vi "HEWH Check For Element Off During Normal Draw.vi"(6 "End of Draw Comparison":bool[][](array[boolean]), 9 "Test Complete":bool, 10 "Debug":bool, 11 "Power State":T1) -> (3 "Cutout after Test Complete":bool, 4 "End of Draw Comparison Output":bool[][](array[boolean]))   [LabVIEW 2023]
uses:
  Type Definitions/HEWH Power Elements.ctl
  Utility/Type Definitions/UTILITY Notifier.ctl
panel:
  out "Index Stop":i32
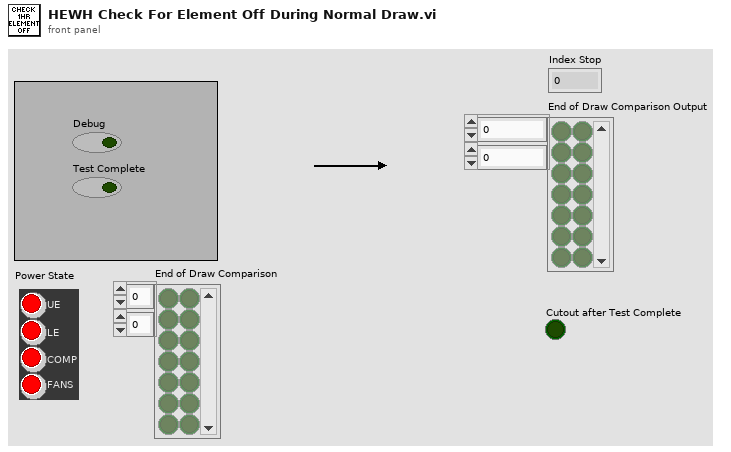
[diagram p1: front panel]
types:
  T1 = typedef "HEWH Power Elements.ctl" = cluster{"UE":bool, "LE":bool, "COMP":bool, "FANS":bool}
  T2 = typedef "UTILITY Notifier.ctl" = enum16{"Set", "Read", "Release Ref"}
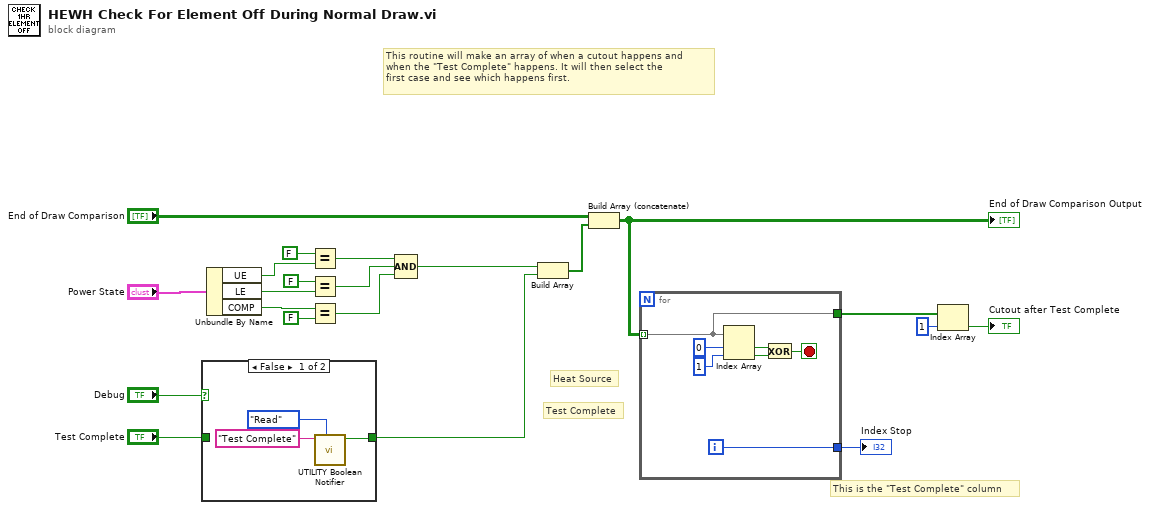
[diagram p0: block diagram]
diagram:
  # "Test Complete"
  # "Heat Source"
  # "This routine will make an array of when a cutout happens and \nwhen the \"Test Complete\" happens. It will then select the \nfirst case and see which happens first."
  # "This is the \"Test Complete\" column"
  n1 = case shown="False" "Debug" {
    tunnel: [w22 w25] -> w10
    tunnel: "Test Complete" -> [_ w25]
    frame False {
      n2 = call "UTILITY Boolean Notifier.vi"("Status"=UTILITY_Notifier."Read", "name (unnamed)"="Test Complete") -> ("latest READ notification"=w22:bool)  [unwired: 8 in, 1 out]
    }
    frame True {
    }
  }
  n3 = Unbundle By Name("Power State") -> ("UE"=w20:bool, "LE"=w19:bool, "COMP"=w18:bool)
  n4 = Equal?(x=FALSE, y=w20) -> (x = y?=w14:bool)
  n5 = Equal?(x=FALSE, y=w19) -> (x = y?=w13:bool)
  n6 = Equal?(x=w18, y=FALSE) -> (x = y?=w12:bool)
  n7 = Compound Arithmetic op=AND(w14, w13, w12) -> (w8:bool)
  n8 = Build Array(w8, w10) -> (w9:bool[])
  n9 = Build Array (concatenate)("End of Draw Comparison", w9) -> (w2:bool[][])
  "End of Draw Comparison Output" <- w2
  n10 = for {
    tunnel: w2 -> [w27] mode=indexing
    tunnel: [w27] -> w7
    tunnel: [w26] -> w4
    i -> [w26]
    stop <- w28 stop-if-true
    n11 = Index Array(array=w27, index #1=0 ("index"), index #2=1 ("index")) -> (element #1=w32:bool, element #2=w31:bool)
    n12 = Exclusive Or(1:w31, 2:w32) -> (0:w28:bool)
  }
  "Index Stop" <- w4
  n13 = Index Array(array=w7, index=1) -> (element=→"Cutout after Test Complete":bool)
